vi "Load and Split Data from File.vi"(0 "Filename":path=path "E:/LabVIEW/Data/Test Data/Subj-Austin_Trial-1_Condition-None.lvm", 5 "Error In":errorcluster) -> (9 "All":dynamicdata(graph), 10 "Sensor 5":dynamicdata(graph), 11 "Mic 1":dynamicdata(graph), 12 "Sensor 6":dynamicdata(graph), 13 "Mic 2":dynamicdata(graph), 14 "Filename Out":path=path "E:/LabVIEW/Data/Test Data/Subj-Austin_Trial-1_Condition-None.lvm" caption="Filename", 15 "Sensor 1":dynamicdata(graph), 16 "Sensor 2":dynamicdata(graph), 17 "Sensor 3":dynamicdata(graph), 18 "Sensor 4":dynamicdata(graph), 19 "Error Out":errorcluster)   [LabVIEW 2019]
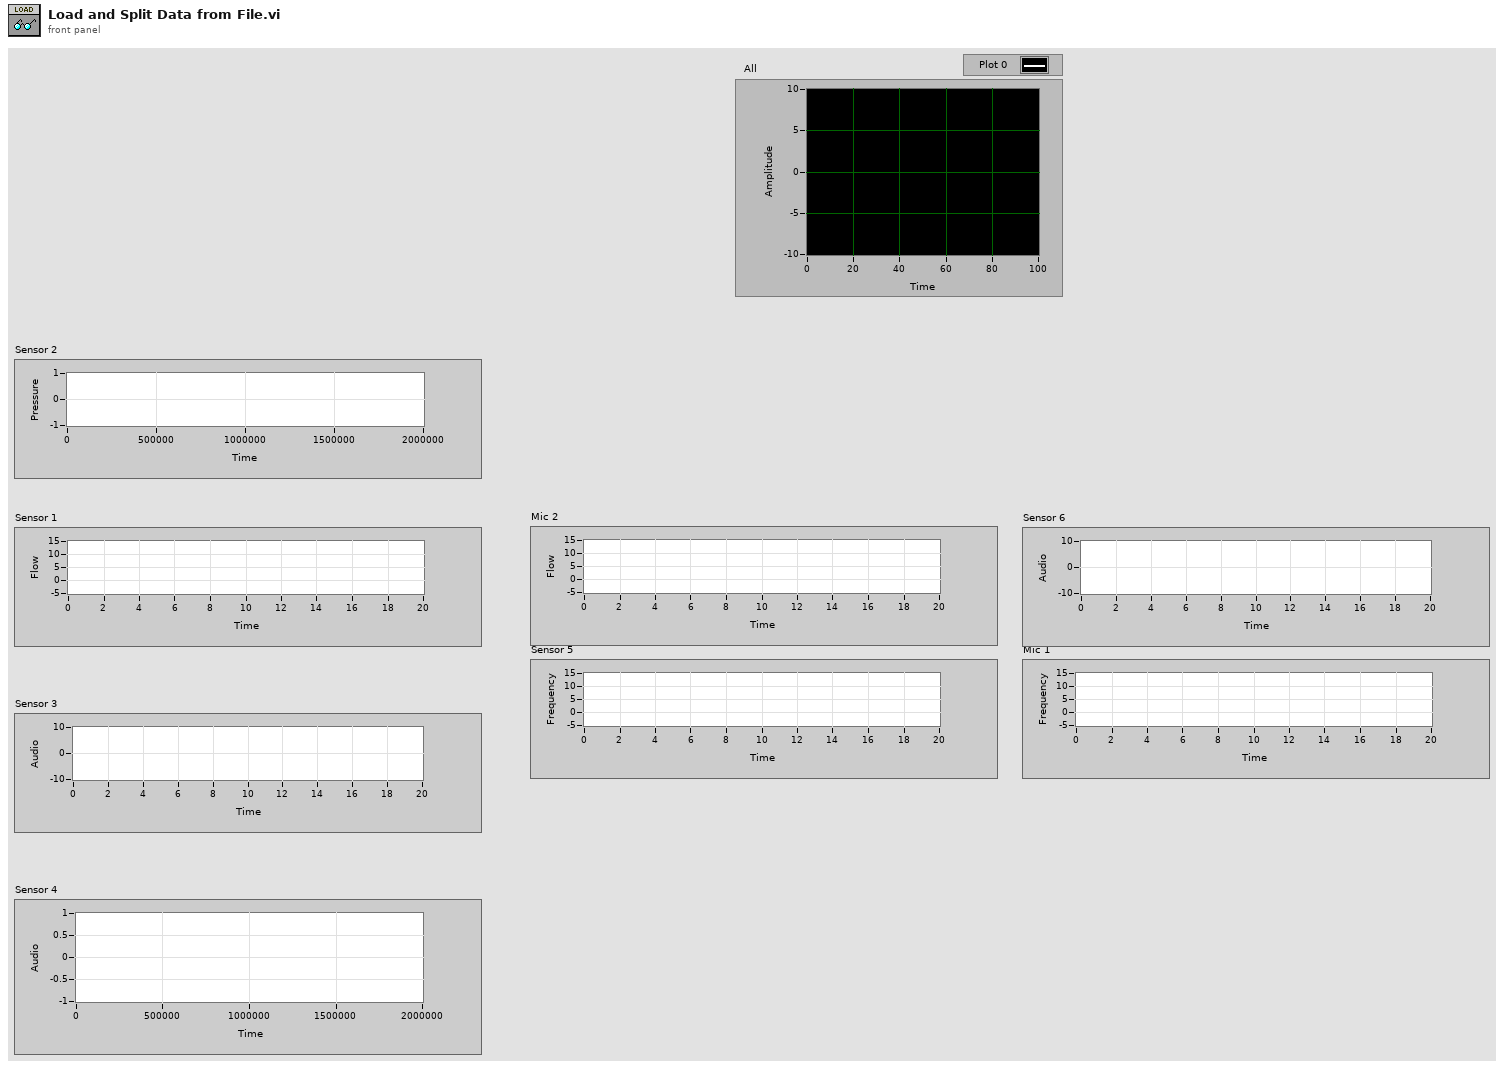
[diagram p1: front panel]
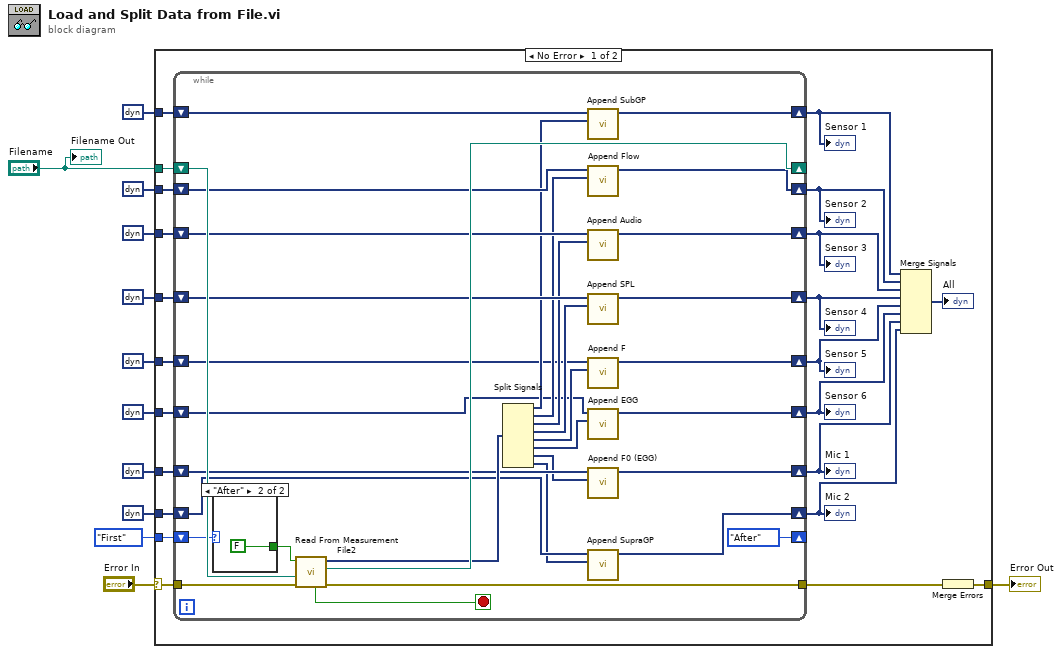
[diagram p0: block diagram]
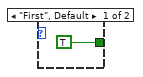
[diagram p2: hidden frame]
diagram:
  n1 = case shown="No Error" "Error In" {
    selector: "Error In" -> [w22 w70]
    tunnel: [w23 w70] -> w11
    tunnel: "Filename" -> [w33 _]
    tunnel: dynamicdata [] ("Waveform Graph") -> [w32 _]
    tunnel: dynamicdata [] ("Waveform Graph") -> [w31 _]
    tunnel: dynamicdata [] ("Waveform Graph") -> [w30 _]
    tunnel: dynamicdata [] ("Waveform Graph") -> [w29 _]
    tunnel: enum16{"First", "After"}."First" -> [w28 _]
    tunnel: dynamicdata [] ("Waveform Graph") -> [w27 _]
    tunnel: dynamicdata [] ("Waveform Graph") -> [w26 _]
    tunnel: dynamicdata [] ("Waveform Graph") -> [w25 _]
    tunnel: dynamicdata [] ("Waveform Graph") -> [w24 _]
    frame No Error {
      n2 = while {
        shift-right: [w67] -> _
        shift-left: w33 -> [w64]
        shift-right: [w55] -> w21
        shift-left: w32 -> [w62]
        shift-right: [w50] -> w20
        shift-left: w31 -> [w61]
        shift-right: [w54] -> w19
        shift-left: w30 -> [w60]
        shift-right: [w51] -> w18
        shift-left: w29 -> [w59]
        shift-right: [enum16{"First", "After"}."After"] -> _
        shift-left: w28 -> [w49]
        shift-right: [w44] -> w17
        shift-left: w27 -> [w45]
        tunnel: w22 -> [w65]
        tunnel: [w66] -> w34
        shift-right: [w43] -> w14
        shift-left: w26 -> [w39]
        shift-right: [w42] -> w16
        shift-left: w25 -> [w38]
        shift-right: [w41] -> w15
        shift-left: w24 -> [w40]
        stop <- w63 stop-if-true
        n3 = case shown="\"After\"" w49 {
          tunnel: [TRUE ("Reset") FALSE ("Reset")] -> w48
          frame "First", Default {
          }
          frame "After" {
          }
        }
        n4 = call "Read From Measurement File2"("error in (no error)"=w65, "Filename"=w64, "Reset"=w48) -> ("error out"=w66:errorcluster, "Filename Out"=w67:path, "Signals"=w52:dynamicdata, "EOF?"=w63:bool)  [unwired: 3 in, 2 out]
        n5 = Split Signals(w52) -> (w58:dynamicdata, w57:dynamicdata, w56:dynamicdata, w53:dynamicdata, w46:dynamicdata, w36:dynamicdata, w35:dynamicdata, w37:dynamicdata)  [unwired: 8 in]
        n6 = call "Append SubGP"("Input Signal B"=w58, "Input Signal A"=w62) -> ("Appended Signals"=w55:dynamicdata)  [unwired: 8 in, 1 out]
        n7 = call "Append Flow"("Input Signal B"=w57, "Input Signal A"=w61) -> ("Appended Signals"=w50:dynamicdata)  [unwired: 8 in, 1 out]
        n8 = call "Append Audio"("Input Signal B"=w56, "Input Signal A"=w60) -> ("Appended Signals"=w54:dynamicdata)  [unwired: 8 in, 1 out]
        n9 = call "Append SPL"("Input Signal B"=w53, "Input Signal A"=w59) -> ("Appended Signals"=w51:dynamicdata)  [unwired: 8 in, 1 out]
        n10 = call "Append F"("Input Signal B"=w46, "Input Signal A"=w45) -> ("Appended Signals"=w44:dynamicdata)  [unwired: 8 in, 1 out]
        n11 = call "Append EGG"("Input Signal B"=w36, "Input Signal A"=w38) -> ("Appended Signals"=w42:dynamicdata)  [unwired: 8 in, 1 out]
        n12 = call "Append F0 (EGG)"("Input Signal B"=w35, "Input Signal A"=w40) -> ("Appended Signals"=w41:dynamicdata)  [unwired: 8 in, 1 out]
        n13 = call "Append SupraGP"("Input Signal B"=w37, "Input Signal A"=w39) -> ("Appended Signals"=w43:dynamicdata)  [unwired: 8 in, 1 out]
      }
      "Sensor 2" <- w20
      "Sensor 1" <- w21
      "Sensor 4" <- w18
      "Sensor 3" <- w19
      "Sensor 5" <- w17
      "Mic 2" <- w14
      "Sensor 6" <- w16
      "Mic 1" <- w15
      n14 = Merge Signals(w21, w20, w19, w18, w17, w16, w15, w14) -> (→"All":dynamicdata)
      n15 = Merge Errors(w34) -> (w23:errorcluster)
    }
    frame Error {
    }
  }
  "Error Out" <- w11
  "Filename Out" <- "Filename"
